vi "TDMS(Write).vi"(8 "error in (no error)":errorcluster caption="错误输入（无错误）", 10 "数据":waveform(dbl)[](array[waveform]), 11 "保存文件名称":string) -> (0 "error out":errorcluster caption="错误输出")   [LabVIEW 2020, in "人体健康监测系统.lvclass"]
uses:
  de3a3521-08cf-4b18-9780-8c738ad00e53.vi
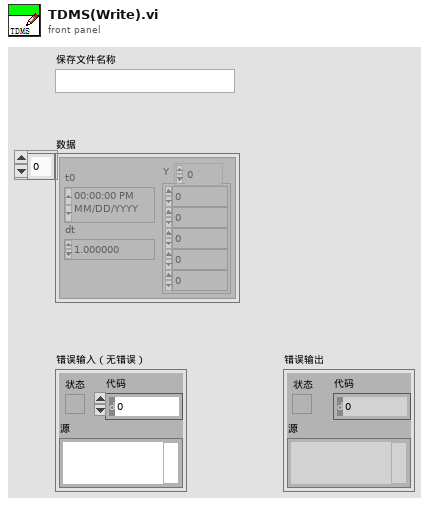
[diagram p1: front panel]
types:
  T1 = enum16{"open", "open or create", "create or replace", "create", "open (read-only)"}
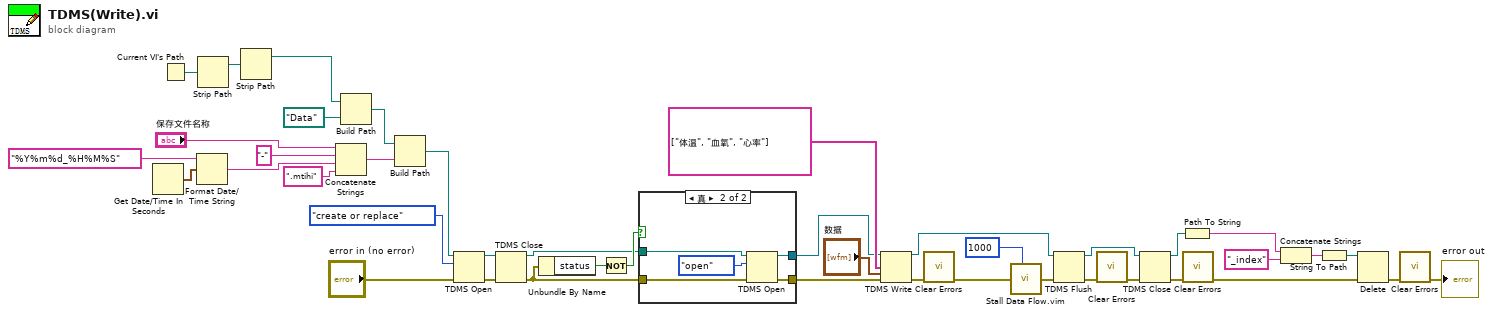
[diagram p0: block diagram]
diagram:
  n1 = Get Date/Time In Seconds() -> (seconds since 1Jan1904=w32:timestamp)
  n2 = Current VI's Path() -> (path=w24:path)
  n3 = Format Date/Time String(time format string (%c)="%Y%m%d_%H%M%S" ("时间格式字符串(%c)"), seconds (now)=w32) -> (date/time string=w29:string)  [unwired: 1 in]
  n4 = Strip Path(path=w24) -> (stripped path=w23:path)  [unwired: 1 out]
  n5 = Strip Path(path=w23) -> (stripped path=w22:path)  [unwired: 1 out]
  n6 = Concatenate Strings("保存文件名称", "-" ("字符串"), w29, ".mtihi" ("字符串")) -> (w27:string)
  n7 = Build Path(base path=w22, name or relative path=path "Data" ("名称或相对路径")) -> (appended path=w20:path)
  n8 = Build Path(base path=w20, name or relative path=w27) -> (appended path=w26:path)
  n9 = TDMS Open(8:"error in (no error)", 10:T1."create or replace" ("操作(0:open)"), 11:w26) -> (0:w34:errorcluster, 3:w35:refnum<k34>)  [unwired: 4 in]
  n10 = TDMS Close(8:w34, 11:w35) -> (0:w17:errorcluster, 3:w18:path)
  n11 = Unbundle By Name(w17) -> ("status"=w33:bool)
  n12 = Not(x=w33) -> (.not. x?=w25:bool)
  n13 = case shown="真" w25 {
    tunnel: [_ w47] -> w19
    tunnel: [w43 w46] -> w16
    tunnel: w18 -> [_ w45]
    tunnel: w17 -> [w43 w44]
    frame False {
    }
    frame True {
      n14 = TDMS Open(8:w44, 10:T1."open" ("操作(0:open)"), 11:w45) -> (0:w46:errorcluster, 3:w47:refnum<k34>)  [unwired: 4 in]
    }
  }
  n15 = TDMS Write(0:w19, 7:string[] ["体温", "血氧", "心率"] ("通道名输入（无标题）"), 9:"数据", 11:w16) -> (4:w41:refnum<k34>, 15:w40:errorcluster)  [unwired: 2 in, 2 out]
  n16 = call <vilib>:"Clear Errors.vi"("error in (no error)"=w40) -> ("error out"=w38:errorcluster)  [unwired: 5 in, 1 out]
  n17 = call "Stall Data Flow.vim"("value in"=w38, "milliseconds to wait"=u32 1000) -> ("value out"=w13:errorcluster)  [unwired: 1 out]
  n18 = TDMS Flush(4:w13, 7:w41) -> (0:w39:errorcluster, 3:w3:refnum<k34>)
  n19 = call <vilib>:"Clear Errors.vi"("error in (no error)"=w39) -> ("error out"=w4:errorcluster)  [unwired: 5 in, 1 out]
  n20 = TDMS Close(8:w4, 11:w3) -> (0:w6:errorcluster, 3:w11:path)
  n21 = Path To String(path=w11) -> (string=w10:string)
  n22 = call <vilib>:"Clear Errors.vi"("error in (no error)"=w6) -> ("error out"=w7:errorcluster)  [unwired: 5 in, 1 out]
  n23 = Concatenate Strings(w10, "_index") -> (w8:string)
  n24 = String To Path(string=w8) -> (path=w5:path)
  n25 = Delete(path (use dialog)=w5, error in=w7) -> (error out=w2:errorcluster)  [unwired: 3 in, 2 out]
  n26 = call <vilib>:"Clear Errors.vi"("error in (no error)"=w2) -> ("error out"=→"error out":errorcluster)  [unwired: 5 in, 1 out]
